vi "Update Device Temperature.vi"(8 "error in (no error)":errorcluster, 10 "Update Temperature Counter":i32, 11 "Message Queue in":refnum<class "Delacor_lib_QMH_Message Queue.lvclass">) -> (0 "error out":errorcluster, 2 "Update Temperature Counter out":i32)   [LabVIEW 2015, in "Tool Module.lvlib"]
doc: "<b>Note:</b> This VI was modified by the <b>Validate DQMH Module</b> tool to turn off automatic error handling."
uses:
  Tool Module.lvlib
  <vilib>/Delacor/Delacor QMH/Libraries/Message Queue_class/Delacor_lib_QMH_Message Queue.lvclass
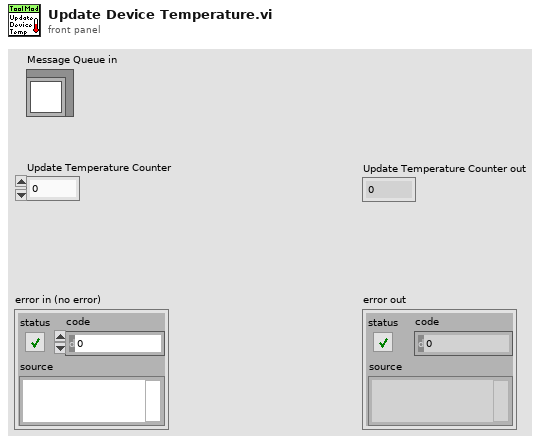
[diagram p1: front panel]
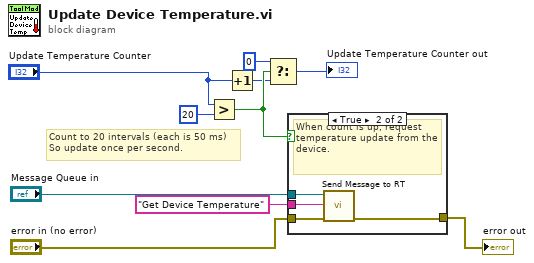
[diagram p0: block diagram]
diagram:
  # "Count to 20 intervals (each is 50 ms)\nSo update once per second."
  n1 = Greater?(x="Update Temperature Counter", y=20) -> (0:w5:bool)
  n2 = Increment(x="Update Temperature Counter") -> (x+1=w3:i32)
  n3 = Select(t=0, s=w5, f=w3) -> (s? t:f=→"Update Temperature Counter out":i32)
  n4 = case shown="True" w5 {
    tunnel: "Message Queue in" -> [_ w15]
    tunnel: "error in (no error)" -> [w11 w14]
    tunnel: "Get Device Temperature" ("Message") -> [_ w13]
    tunnel: [w11 w12] -> w4
    frame False {
    }
    frame True {
      # "When count is up, request temperature update from the device."
      n5 = call "Send Message to RT.vi"("error in (no error)"=w14, "Message"=w13, "Message Queue in"=w15) -> ("error out"=w12:errorcluster)  [unwired: 7 in, 1 out]
    }
  }
  "error out" <- w4
